vi "disableWatchdog.vi"(9 "Fault in":bool, 10 "FPGA VI Reference In":refnum<k20>) -> (1 "Fault out":bool, 2 "FPGA VI Reference Out":refnum<k20>)   [LabVIEW 2017]
uses:
  <vilib>/Utility/error.llb/Error Cluster From Error Code.vi
  <vilib>/rvi/errors/niLvFpgaAdjustHostInterfaceError.vi
  <vilib>/rvi/interface/nirviReadWriteControl/nirviReadWriteControl.xnode
  NiFpgaLv.dll
  <vilib>/rvi/interface/Simulation/niFpgaSimulationCallBeginRW.vi
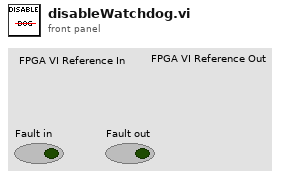
[diagram p1: front panel]
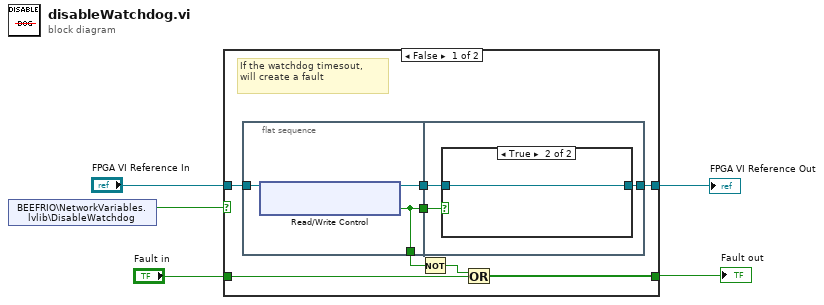
[diagram p0: block diagram]
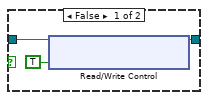
[diagram p2: hidden frame]
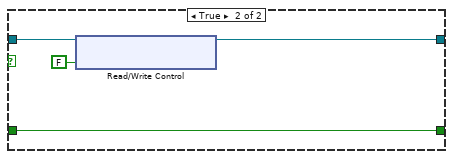
[diagram p3: hidden frame]
diagram:
  n1 = shared-variable "BEEFRIO\\NetworkVariables.lvlib\\DisableWatchdog"() -> (w5:bool)  [unwired: 1 in, 1 out]
  n2 = case shown="False" w5 {
    tunnel: [w9 w27] -> w1
    tunnel: "FPGA VI Reference In" -> [w13 w26]
    tunnel: [w11 w25] -> w3
    tunnel: "Fault in" -> [w10 w25]
    frame False {
      # "If the watchdog timesout,\nwill create a fault"
      n3 = flat-sequence {
        tunnel: w13 -> [w16]
        tunnel: [w14] -> w12
        tunnel: [w15] -> w8
        tunnel: [w14] -> w7
        tunnel: [w18] -> w9
        tunnel: w8 -> [w19]
        tunnel: w7 -> [w17]
        frame #0 {
          n4 = xnode "Read/Write Control"("FPGA VI Reference In"=w16) -> ("FPGA VI Reference Out"=w15:refnum<k20>, "Enable RT Watchdog"=w14:bool)  [unwired: 1 in, 1 out]
        }
        frame #1 {
          n5 = case shown="True" w17 {
            tunnel: w19 -> [w22 w23]
            tunnel: [w21 w23] -> w18
            frame False {
              n6 = xnode "Read/Write Control"("FPGA VI Reference In"=w22, "Enable RT Watchdog"=TRUE) -> ("FPGA VI Reference Out"=w21:refnum<k20>)  [unwired: 1 in, 1 out]
            }
            frame True {
            }
          }
        }
      }
      n7 = Not(x=w12) -> (.not. x?=w6:bool)
      n8 = Or(x=w6, y=w10) -> (x .or. y?=w11:bool)
    }
    frame True {
      n9 = xnode "Read/Write Control"("FPGA VI Reference In"=w26, "Enable RT Watchdog"=FALSE) -> ("FPGA VI Reference Out"=w27:refnum<k20>)  [unwired: 1 in, 1 out]
    }
  }
  "Fault out" <- w3
  "FPGA VI Reference Out" <- w1
